vi "Register for File Close Event.vi"(8 "error in (no error)":errorcluster, 9 "User Data":variant, 10 "Callback":refnum<vi>, 11 "Segmented Log in":refnum<class "Segmented Log.lvclass">) -> (0 "error out":errorcluster, 3 "Segmented Log out":refnum<class "Segmented Log.lvclass">)   [LabVIEW 2015, in "Segmented Log.lvclass"]
uses:
  Segmented Log.lvclass
  Segmented Log.lvclass/Segmented Log.ctl
  File Close Event Registration.ctl
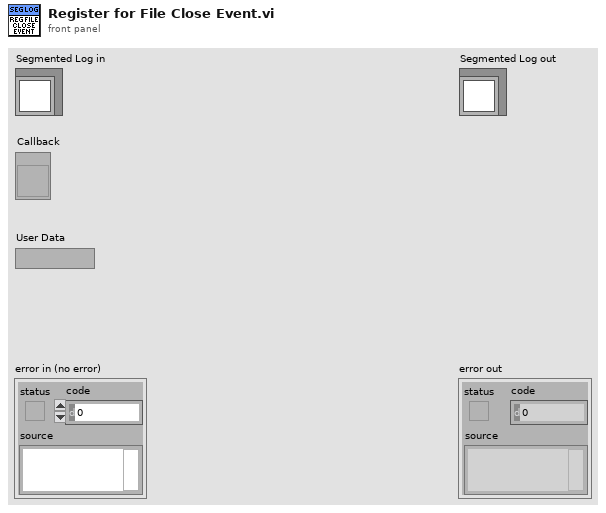
[diagram p1: front panel]
types:
  T1 = typedef "Segmented Log.lvclass/File Close Event Registration.ctl" = cluster{"Callback":refnum<vi>, "User Data":variant}
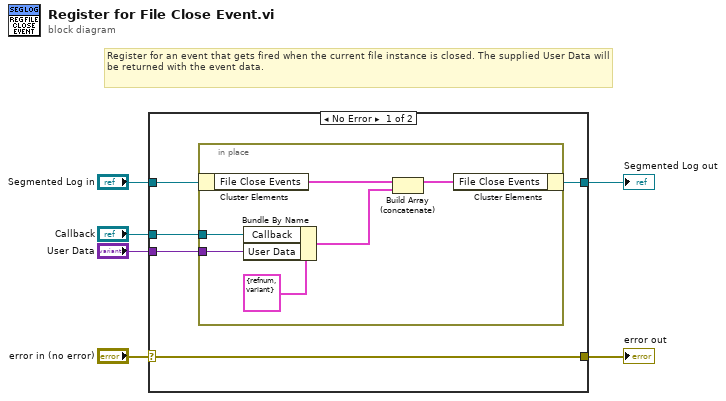
[diagram p0: block diagram]
diagram:
  # "Register for an event that gets fired when the current file instance is closed. The supplied User Data will be returned with the event data."
  n1 = case shown="No Error" "error in (no error)" {
    selector: "error in (no error)" -> [w9 w19]
    tunnel: [w9 w19] -> w5
    tunnel: [w10 w18] -> w3
    tunnel: "Segmented Log in" -> [w11 w18]
    tunnel: "Callback" -> [w8 _]
    tunnel: "User Data" -> [w7 _]
    frame No Error {
      n2 = in-place {
        in-place-border: w8 -> [w14]
        in-place-border: w7 -> [w12]
        n3 = in-place-cluster #1(w11) -> ("File Close Events"=w17:T1[])
        n4 = Bundle By Name(cluster=T1 {"Callback"=refnum, "User Data"=variant} ("File Close Event Registration"), "Callback"=w14, "User Data"=w12) -> (w13:T1)
        n5 = Build Array (concatenate)(w17, w13) -> (w16:T1[])
        n6 = in-place-cluster #1("File Close Events"=w16) -> (w10:refnum<class "Segmented Log.lvclass">)
      }
    }
    frame Error {
    }
  }
  "error out" <- w5
  "Segmented Log out" <- w3
